vi "NIP Data.vi"(10 "index (row)":i32, 11 "file path (dialog if empty)":path) -> (2 "Data":string[][](array[string]), 3 "file path (dialog if empty) 2":path)   [LabVIEW 2015]
uses:
  <vilib>/Utility/file.llb/Read Delimited Spreadsheet (string).vi
  Galobal variable_TI.vi
panel:
  out "Write Data":string[](array[string])
  out "output array":string[][](array[string])
  out "error out":errorcluster
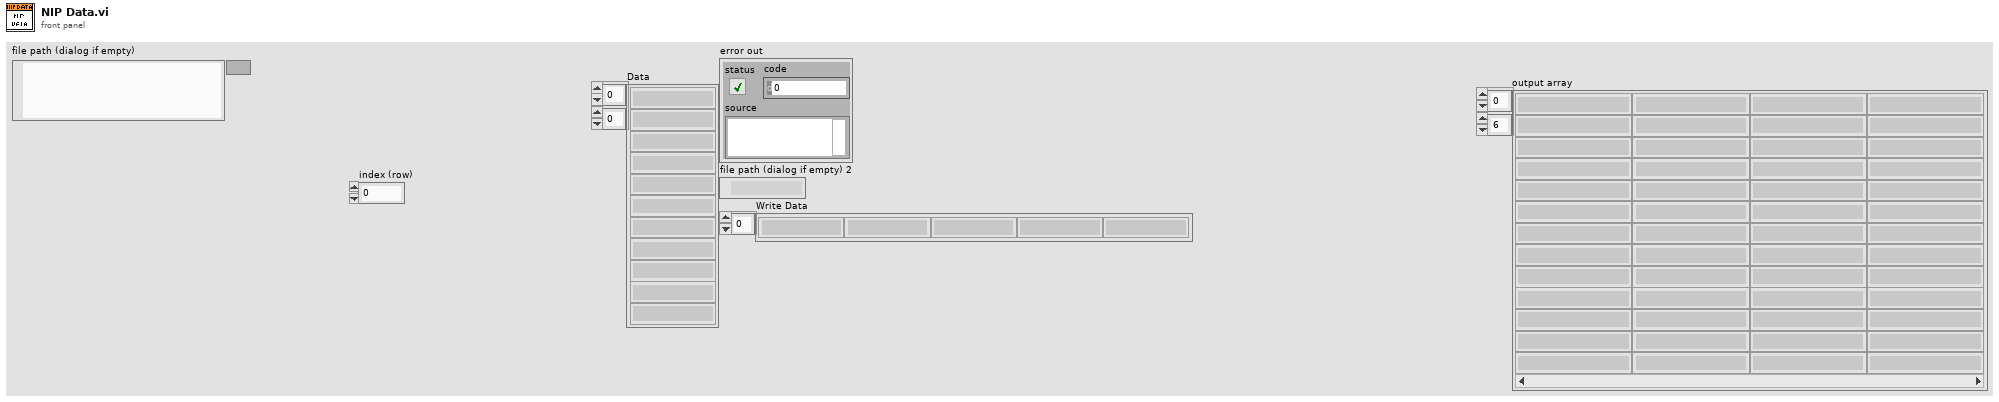
[diagram p1: front panel]
types:
  T1 = cluster{"To-A":timestamp, "From-A":timestamp, "From-B":timestamp, "To-B":timestamp, "From-C 1":timestamp, "To-C 1":timestamp, "From-C 2":timestamp, "To-C 2":timestamp, "Shift":string}
  T2 = cluster{"To-A":timestamp, "From-A":timestamp, "From-B":timestamp, "To-B":timestamp, "From-C 1":timestamp, "To-C 1":timestamp, "From-C 2":timestamp, "To-C 2":timestamp}
  T3 = cluster{"No. Fail Coun t":string, "Rework Status Count 0\\1":string, "NA Count Max =3 ":string, "Testesd Count  0/1":string, "Error code":string}
  T4 = cluster{"Stn Name":string, "date":string, "time":string, "Operator id":string, "Shift":string, "Error Code":string, "Fail count":string, "Rework":string, "NA":string, "Tested":string}
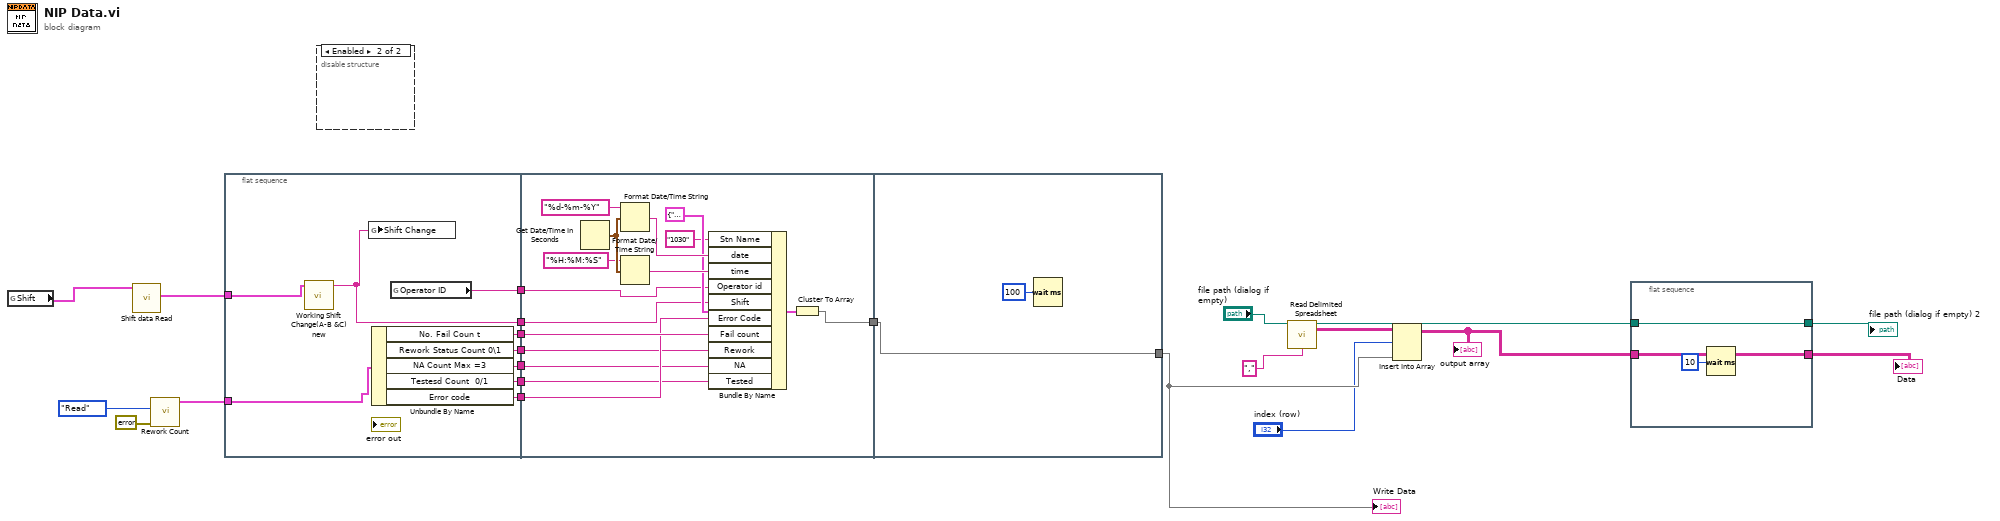
[diagram p0: block diagram]
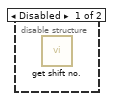
[diagram p2: hidden frame]
diagram:
  n1 = global read "Galobal variable_TI.vi" "Shift"() -> (w15:T1)
  n2 = call "Shift data Read.vi"("input cluster"=w15) -> ("output cluster"=w16:T2)  [unwired: 10 in]
  n3 = call "Rework Count.vi"("error in"=errorcluster {"status"=FALSE, "code"=0, "source"=""}, "Read /Write"=enum16{"Write", "Read"}."Read") -> ("data"=w11:T3)  [unwired: 8 in, 1 out]
  n4 = flat-sequence {
    tunnel: [w31] -> w22
    tunnel: [w30] -> w21
    tunnel: [w29] -> w20
    tunnel: [w28] -> w19
    tunnel: [w27] -> w18
    tunnel: w16 -> [w26]
    tunnel: [w25] -> w14
    tunnel: w11 -> [w24]
    tunnel: [w23] -> w1
    tunnel: w22 -> [w39]
    tunnel: w21 -> [w38]
    tunnel: w20 -> [w37]
    tunnel: w19 -> [w36]
    tunnel: w18 -> [w35]
    tunnel: [w34] -> w17
    tunnel: w14 -> [w33]
    tunnel: w1 -> [w32]
    tunnel: w17 -> [w48]
    tunnel: [w48] -> w8
    frame #0 {
      n5 = call "Working Shift Change(A-B &C) new.vi"("input cluster"=w26) -> ("Shift Change"=w25:string)  [unwired: 10 in]
      n6 = global write "Galobal variable_TI.vi" "Shift Change"(w25) -> ()
      n7 = Unbundle By Name(w24) -> ("No. Fail Coun t"=w31:string, "Rework Status Count 0\\1"=w29:string, "NA Count Max =3"=w28:string, "Testesd Count  0/1"=w27:string, "Error code"=w30:string)
      n8 = global read "Galobal variable_TI.vi" "Operator ID"() -> (w23:string)
    }
    frame #1 {
      n9 = Get Date/Time In Seconds() -> (seconds since 1Jan1904=w45:timestamp)
      n10 = Format Date/Time String(time format string (%c)="%d-%m-%Y", seconds (now)=w45) -> (date/time string=w46:string)  [unwired: 1 in]
      n11 = Format Date/Time String(time format string (%c)="%H:%M:%S", seconds (now)=w45) -> (date/time string=w43:string)  [unwired: 1 in]
      n12 = Bundle By Name(cluster=T4 {"Stn Name"="", "date"="", "time"="", "Operator id"="", "Shift"="", "Error Code"="", "Fail count"="", "Rework"="", "NA"="", "Tested"=""} ("Write Data"), "Stn Name"="1030", "date"=w46, "time"=w43, "Operator id"=w32, "Shift"=w33, "Error Code"=w38, "Fail count"=w39, "Rework"=w37, "NA"=w36, "Tested"=w35) -> (w42:T4)
      n13 = Cluster To Array(cluster=w42) -> (array=w34:string[])
    }
    frame #2 {
      n14 = Wait (ms)(milliseconds to wait=u32 100) -> ()  [unwired: 1 out]
    }
  }
  n15 = disable-structure shown="Enabled" {
    frame Disabled {
      n16 = call "get shift no..vi"() -> ()  [unwired: 11 in, 1 out]
    }
    frame Enabled {
    }
  }
  n17 = call-poly <vilib>:"Read Delimited Spreadsheet.vi"("file path (dialog if empty)"="file path (dialog if empty)", "delimiter (\\t)"="," ("delimiter (\\t)")) -> ("new file path (Not A Path if cancelled)"=w6:path, "all rows"=w10:string[][])  [unwired: 8 in, 4 out]
  n18 = Insert Into Array(array=w10, index (row)="index (row)", new element=w8) -> (w7:string[][])  [unwired: 1 in]
  "output array" <- w7
  n19 = flat-sequence {
    tunnel: w7 -> [w50]
    tunnel: w6 -> [w52]
    tunnel: [w52] -> w5
    tunnel: [w50] -> w4
    frame #0 {
      n20 = Wait (ms)(milliseconds to wait=u32 10) -> ()  [unwired: 1 out]
    }
  }
  "file path (dialog if empty) 2" <- w5
  "Data" <- w4
  "Write Data" <- w8
